vi "SwissSPAD Live_Get FPGA Status String.vi"(8 "error in (no error)":errorcluster, 9 "Init Communication Outcome":T1, 11 "SwissSPAD Live Internal Variables in":T2 {"# Acquisitions" min=1; "Image Binning Options"."Y Bin" min=1; "Image Binning Options"."X Bin" min=1}) -> (0 "error out":errorcluster, 1 "Device Info String":string, 3 "SwissSPAD Live Internal Variables out":T2 {"# Acquisitions" min=1; "Image Binning Options"."Y Bin" min=1; "Image Binning Options"."X Bin" min=1}, 5 "Top FPGA Status":bool, 7 "Bottom FPGA Status":bool)   [LabVIEW 2021]
uses:
  SwissSPAD Live_Internal Variables.ctl
  D:/UCLA Thinkpad Google Drive/LabVIEW 2021 SP1/builds/SwissSPAD Live Distribution/Opal Kelly/C# Wrapper/v5.0.2/libFrontPanel-csharp.dll
  Opal Kelly/C# Wrapper/v5.0.2/libFrontPanel-csharp.dll
  <vilib>/vision/Image Controls.llb/IMAQ Image.ctl
  SwissSPAD Live_Image ROI Information.ctl
  Phasor/Image Binning Options.ctl
  SwissSPAD Live_SSx PCB Version.ctl
  SwissSPAD Live_Init Communication Outcome.ctl
  Opal Kelly/C# Wrapper/okFrontPanelC#Wrapper.lvlib
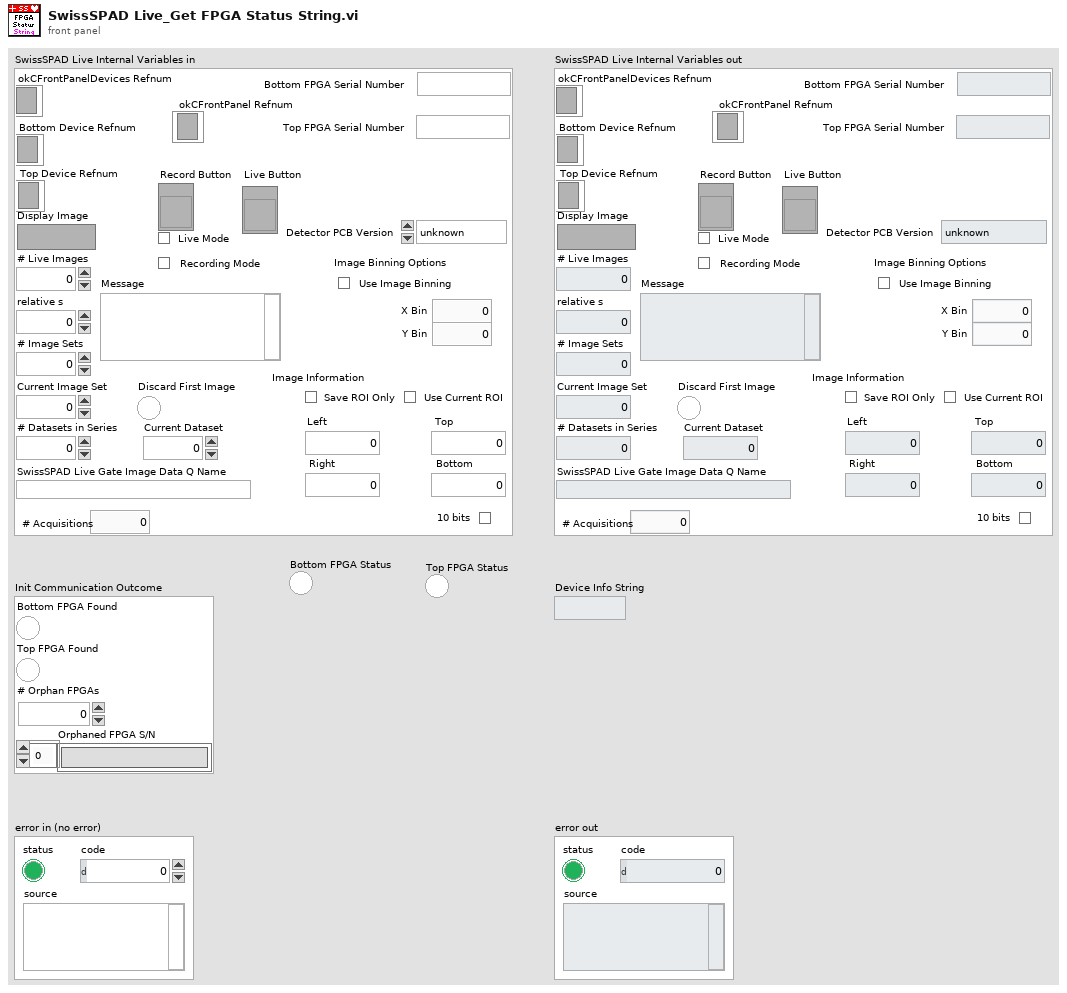
[diagram p1: front panel]
types:
  T1 = typedef "SwissSPAD Live_Init Communication Outcome.ctl" = cluster{"Bottom FPGA Found":bool, "Top FPGA Found":bool, "# Orphan FPGAs":i32, "Orphaned FPGA S/N":string[]}
  T2 = typedef "SwissSPAD Live_Internal Variables.ctl" = cluster{"okCFrontPanelDevices Refnum":refnum<k24>, "Bottom Device Refnum":refnum<k24>, "Display Image":T3, "# Live Images":i32, "relative s":dbl, "# Image Sets":i32, "Message":string, "Current Image Set":i32, "# Datasets in Series":i32, "Current Dataset":i32, "Live Mode":bool, "Recording Mode":bool, "Record Button":refnum<vi>, "\nLive Button":refnum<vi>, "SwissSPAD Live Gate Image Data Q Name":string, "Discard First Image":bool, "Image Information":T4, "Image Binning Options":T5, "Bottom FPGA Serial Number":string, "Detector PCB Version":T6, "# Acquisitions":u32, "10 bits":bool, "Top FPGA Serial Number":string, "Top Device Refnum":refnum<k24>, "okCFrontPanel Refnum":refnum<k24>}
  T3 = typedef "IMAQ Image.ctl" = refnum<image>
  T4 = typedef "SwissSPAD Live_Image ROI Information.ctl" = cluster{"Save ROI Only":bool, "Left":u16, "Top":u16, "Right":u16, "Bottom":u16, "Use Current ROI":bool}
  T5 = typedef "Image Binning Options.ctl" = cluster{"Use Image Binning":bool, "X Bin":i32, "Y Bin":i32}
  T6 = typedef "SwissSPAD Live_SSx PCB Version.ctl" = enum16{"unknown", "SS2 PCB1", "SS2 PCB2", "SS3 PCB1"}
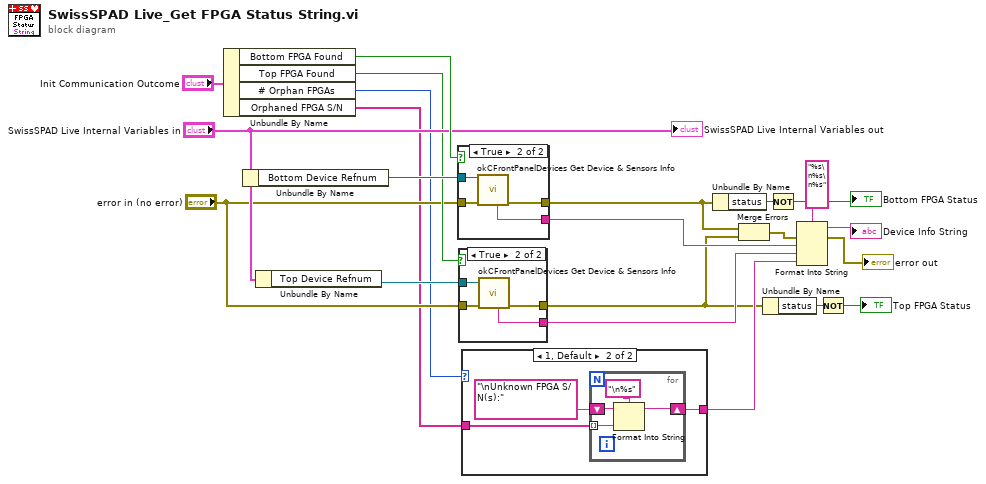
[diagram p0: block diagram]
diagram:
  n1 = Unbundle By Name("Init Communication Outcome") -> ("Bottom FPGA Found"=w21:bool, "Top FPGA Found"=w18:bool, "# Orphan FPGAs"=w15:i32, "Orphaned FPGA S/N"=w14:string[])
  n2 = Unbundle By Name("SwissSPAD Live Internal Variables in") -> ("Bottom Device Refnum"=w20:refnum<k24>)
  n3 = Unbundle By Name("SwissSPAD Live Internal Variables in") -> ("Top Device Refnum"=w17:refnum<k24>)
  n4 = case shown="True" w21 {
    tunnel: "error in (no error)" -> [w23 w27]
    tunnel: [w23 w26] -> w6
    tunnel: w20 -> [_ w25]
    tunnel: [_ w24] -> w13
    frame False {
    }
    frame True {
      n5 = call "okCFrontPanelDevices Get Device & Sensors Info.vi"("error in (no error)"=w27, "okCFrontPanel Device Refnum"=w25) -> ("error out"=w26:errorcluster, "Device Info String"=w24:string)  [unwired: 5 in, 3 out]
    }
  }
  n6 = case shown="True" w18 {
    tunnel: "error in (no error)" -> [w28 w32]
    tunnel: [w28 w31] -> w2
    tunnel: w17 -> [_ w30]
    tunnel: [_ w29] -> w12
    frame False {
    }
    frame True {
      n7 = call "okCFrontPanelDevices Get Device & Sensors Info.vi"("error in (no error)"=w32, "okCFrontPanel Device Refnum"=w30) -> ("error out"=w31:errorcluster, "Device Info String"=w29:string)  [unwired: 5 in, 3 out]
    }
  }
  n8 = case shown="1, Default" w15 {
    tunnel: w14 -> [_ w35]
    tunnel: [_ w33] -> w11
    frame 0 {
    }
    frame 1, Default {
      n9 = for {
        tunnel: w35 -> [w39] mode=indexing
        shift-right: [w38] -> w33
        shift-left: "\nUnknown FPGA S/N(s):" -> [w37]
        n10 = Format Into String(format string="\n%s", initial string=w37, w39) -> (resulting string=w38:string)  [unwired: 1 in, 1 out]
      }
    }
  }
  n11 = Unbundle By Name(w6) -> ("status"=w5:bool)
  n12 = Merge Errors(w6, w2) -> (w7:errorcluster)
  n13 = Unbundle By Name(w2) -> ("status"=w3:bool)
  n14 = Not(x=w5) -> (.not. x?=→"Bottom FPGA Status":bool)
  n15 = Format Into String(format string="%s\n%s\n%s", error in=w7, w13, w12, w11) -> (resulting string=→"Device Info String":string, error out=→"error out":errorcluster)  [unwired: 1 in]
  n16 = Not(x=w3) -> (.not. x?=→"Top FPGA Status":bool)
  "SwissSPAD Live Internal Variables out" <- "SwissSPAD Live Internal Variables in"
